vi "Update Distance and Angle to Wall Using Lidar.vi"(10 "Current State":T1=enum."Follow Wall", 11 "Wall Left?":bool=TRUE) -> (3 "OH SHIT NO LIDAR DATA!!!":bool)   [LabVIEW 2017]
uses:
  state-manager/State.ctl
  Globals/Pose.vi
panel:
  out "XY Graph":cluster{dbl[], dbl[]}(graph)
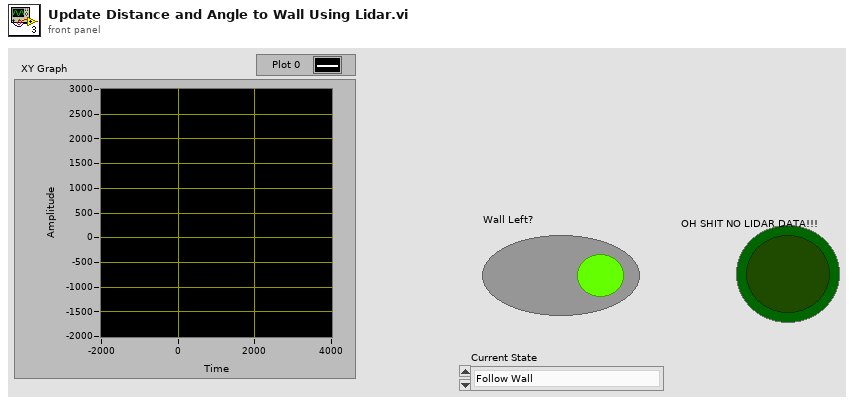
[diagram p1: front panel]
types:
  T1 = typedef "State.ctl" = enum16{"Wait", "Recenter", "Follow Wall", "Zig Zag", "Ramp", "Cross Rough Terrain", "Stagger Stop", "Obstacle Avoidance"}
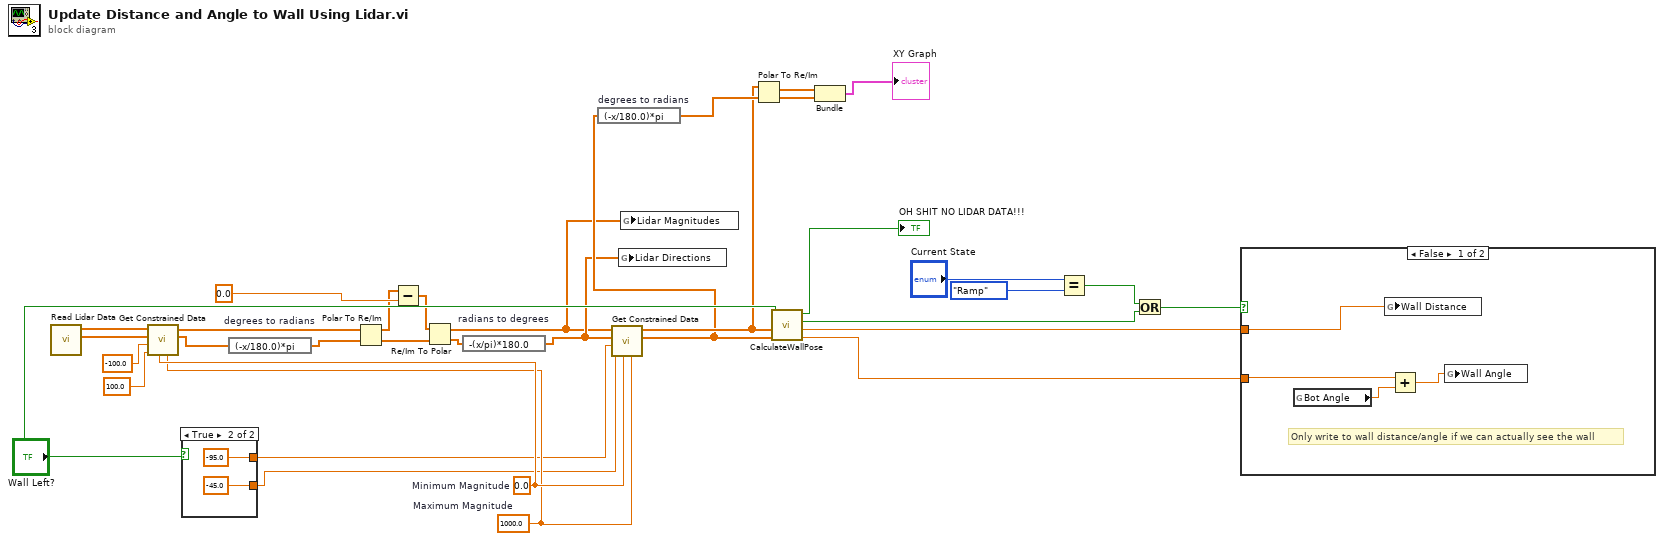
[diagram p0: block diagram]
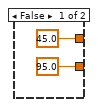
[diagram p3: hidden frame]
diagram:
  w29 = 1000.0  # Maximum Magnitude
  w30 = 0.0  # Minimum Magnitude
  n1 = call "Read Lidar Data.vi"() -> ("Direction"=w16:dbl[], "Magnitude"=w20:dbl[])  [unwired: 9 in, 1 out]
  n2 = call "Get Constrained Data.vi"("Maximum Magnitude"=w29, "Minimum Magnitude"=w30, "Maximum Angle (rad)"=100.0 ("Maximum Angle (DEG)"), "Minimum Angle (rad)"=-100.0 ("Minimum Angle (DEG)"), "Lidar Directions (rad)"=w16, "Lidar Magnitudes"=w20) -> ("Constrained Angles"=w10:dbl[], "Constrained Magnitudes"=w8:dbl[])  [unwired: 4 in]
  n3 = case shown="True" "Wall Left?" {
    tunnel: [45.0 -95.0] -> w12
    tunnel: [95.0 -45.0] -> w11
    frame False {
    }
    frame True {
    }
  }
  n4 = expression code="(-x/180.0)*pi" "degrees to radians"(w10) -> (w9:dbl[])
  n5 = Polar To Re/Im(2:w9, 3:w8) -> (0:w1:dbl[], 1:w2:dbl[])
  n6 = Subtract(x=w2, y=0.0 ("Maximum Angle (DEG)")) -> (x-y=w3:dbl[])
  n7 = Re/Im To Polar(2:w1, 3:w3) -> (0:w6:dbl[], 1:w4:dbl[])
  n8 = expression code="-(x/pi)*180.0" "radians to degrees"(w6) -> (w5:dbl[])
  n9 = call "Get Constrained Data.vi"("Maximum Magnitude"=w29, "Minimum Magnitude"=w30, "Maximum Angle (rad)"=w11, "Minimum Angle (rad)"=w12, "Lidar Directions (rad)"=w5, "Lidar Magnitudes"=w4) -> ("Constrained Angles"=w13:dbl[], "Constrained Magnitudes"=w14:dbl[])  [unwired: 4 in]
  n10 = expression code="(-x/180.0)*pi" "degrees to radians"(w13) -> (w15:dbl[])
  n11 = global write "Pose.vi" "Lidar Directions"(w5) -> ()
  n12 = global write "Pose.vi" "Lidar Magnitudes"(w4) -> ()
  n13 = Polar To Re/Im(2:w15, 3:w14) -> (0:w17:dbl[], 1:w18:dbl[])
  n14 = call "CalculateWallPose.vi"("Lidar Angles"=w13, "Lidar Magnitude"=w14, "Wall Left?"="Wall Left?") -> ("Angle to Wall"=w27:dbl, "Distance to Wall"=w26:dbl, "Can't see wall"=w23:bool, "OH SHIT NO LIDAR DATA!!!"=→"OH SHIT NO LIDAR DATA!!!":bool)  [unwired: 5 in]
  n15 = Bundle(w18, w17) -> (→"XY Graph":cluster{dbl[], dbl[]})  [unwired: 1 in]
  n16 = Equal?(x="Current State", y=State."Ramp") -> (x = y?=w22:bool)
  n17 = Or(x=w22, y=w23) -> (x .or. y?=w21:bool)
  n18 = case shown="False" w21 {
    tunnel: w27 -> [w40 _]
    tunnel: w26 -> [w39 _]
    frame False {
      # "Only write to wall distance/angle if we can actually see the wall"
      n19 = global read "Pose.vi" "Bot Angle"() -> (w41:dbl)
      n20 = global write "Pose.vi" "Wall Distance"(w39) -> ()
      n21 = Add(x=w40, y=w41) -> (x+y=w38:dbl)
      n22 = global write "Pose.vi" "Wall Angle"(w38) -> ()
    }
    frame True {
    }
  }
